vi "Frames to AVI.vi"(0 "Image directory":path=path "C:/Test images", 1 "AVI output path":path=path "C:/Test.avi", 2 "Frames Per Second":u32=1, 3 "Quality":i32=1000, 4 "Format qualifier":string="*.jpg") -> (5 "Images used":string[](array[string]))   [LabVIEW 2014]
panel:
  out "Image":T1(plugin-control)
  out "Error Out":errorcluster
  in  "Codec":string="Microsoft Video 1"
  # "PN 10/12/2014"
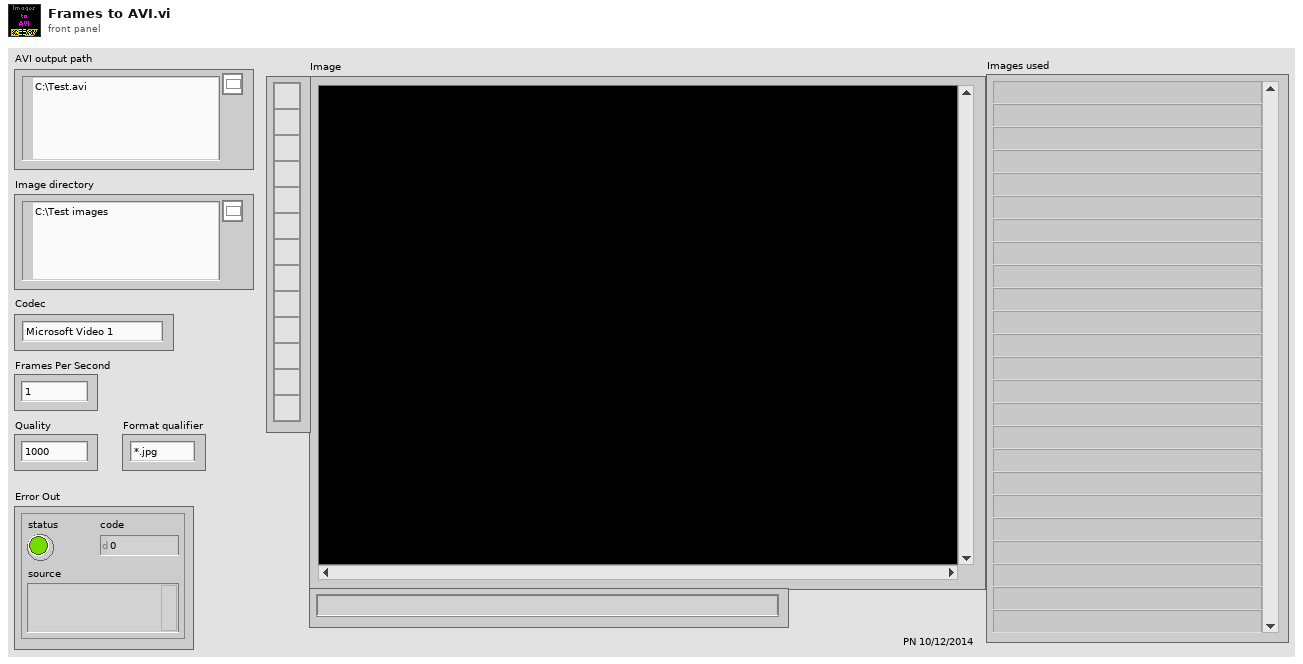
[diagram p1: front panel]
types:
  T1 = typedef "IMAQ Image.ctl" = refnum<image>
  T2 = typedef "Image Type" = u32
  T3 = typedef "IMAQ AVI2 Refnum.ctl" = refnum<k20>
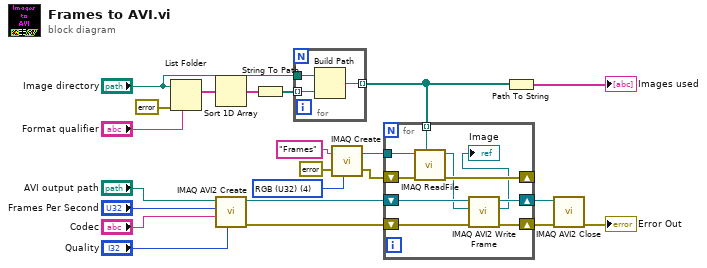
[diagram p0: block diagram]
diagram:
  w1 = T2 4 items=["Grayscale (U8)", "Grayscale (I16)", "Grayscale (SGL)", "Complex (CSG)", "RGB (U32)", "HSL (U32)", "RGB (U64)", "Grayscale (U16)"] ("Image Type")
  n1 = List Folder(path="Image directory", pattern="Format qualifier", error in=errorcluster {"status"=FALSE, "code"=0, "source"=""}) -> (filenames=w3:string[])  [unwired: 1 in, 3 out]
  n2 = Sort 1D Array(array=w3) -> (sorted array=w2:string[])
  n3 = call "IMAQ AVI2 Create"("Quality"="Quality", "Codec"="Codec", "Frames Per Second"="Frames Per Second", "AVI Path"="AVI output path") -> ("error out"=w18:errorcluster, "AVI Refnum"=w15:T3)  [unwired: 6 in]
  n4 = String To Path(string=w2) -> (path=w12:path[])
  n5 = for {
    tunnel: w12 -> [w25] mode=indexing
    tunnel: "Image directory" -> [w24]
    tunnel: [w23] -> w6 mode=indexing
    n6 = Build Path(base path=w24, name or relative path=w25) -> (appended path=w23:path)
  }
  n7 = call "IMAQ Create"("Image Name"="Frames", "Image Type"=w1, "error in (no error)"=errorcluster {"status"=FALSE, "code"=0, "source"=""}) -> ("New Image"=w9:T1, "error out"=w10:errorcluster)  [unwired: 2 in]
  n8 = for {
    shift-right: [w34] -> w17
    shift-left: w18 -> [w35]
    shift-right: [w33] -> w16
    shift-left: w15 -> [w29]
    shift-right: [w31] -> _
    shift-left: w10 -> [w32]
    tunnel: w6 -> [w30] mode=indexing
    tunnel: w9 -> [w27]
    n9 = call "IMAQ ReadFile"("File Path"=w30, "error in (no error)"=w32, "Image"=w27) -> ("error out"=w31:errorcluster, "Image Out"=w28:T1)  [unwired: 4 in, 3 out]
    n10 = call "IMAQ AVI2 Write Frame"("error in (no error)"=w35, "Image"=w28, "AVI Refnum"=w29) -> ("error out"=w34:errorcluster, "Image Out (duplicate)"=→"Image":T1, "AVI Refnum (duplicate)"=w33:T3)  [unwired: 6 in]
  }
  n11 = Path To String(path=w6) -> (string=→"Images used":string[])
  n12 = call "IMAQ AVI2 Close"("error in (no error)"=w17, "AVI Refnum"=w16) -> ("error out"=→"Error Out":errorcluster)  [unwired: 9 in]
